vi "KalmanFilterLatencyComp_FindClosestMeasurement.vi"(9 "TimeStamp_Sec":dbl, 11 "in KalmanFilterLatencyCompensator":T1) -> (0 "NotFound":bool, 3 "Index":i32)   [LabVIEW 2019, in "Trajectory_Library.lvlib"]
doc: "An internal function that finds the item in the Past Observer Snapshot list with the timestamp closest to the one passed as an input.\n\nInputs:\n - inKalmanFilterLatencyCompensator -- Data cluster\n - TimeStamp_Sec -- Relative robot timestamp of the item to find (Seconds)\n\nOutputs:\n - Index -- Integer index to the closest entry\n - NotFound -- Boolean, whose value is TRUE if the closest entry was not found."
uses:
  Trajectory_Library.lvlib
  <vilib>/Analysis/Matrix/Datatypes/RealMatrix.ctl
  <vilib>/Analysis/Matrix/NI_Matrix.lvlib
  TypeDef/OBSERVER_SNAPSHOT.ctl
  TypeDef/OBSERVER_SNAP_LIST_ITEM.ctl
  TypeDef/KALMAN_FILTER_LATENCY_COMP.ctl
panel:
  # "<Statess,1>"
  # "<States, States>"
  # "<Inputs, 1>"
  # "<Outputs,  1>"
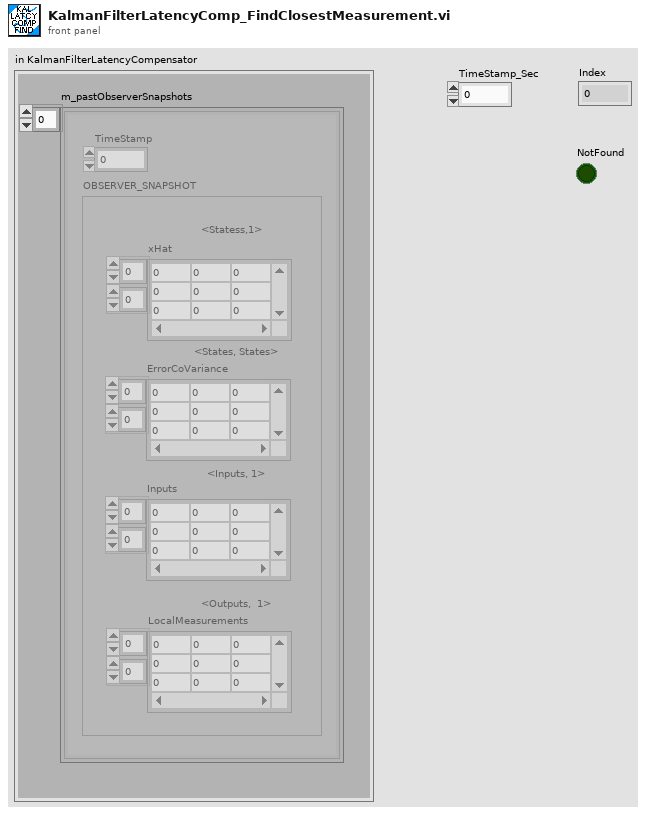
[diagram p1: front panel]
types:
  T1 = typedef "Trajectory_Library.lvlib/KALMAN_FILTER_LATENCY_COMP.ctl" = cluster{"m_pastObserverSnapshots ":T2[]}
  T2 = typedef "Trajectory_Library.lvlib/OBSERVER_SNAP_LIST_ITEM.ctl" = cluster{"TimeStamp":dbl, "OBSERVER_SNAPSHOT":T3}
  T3 = typedef "Trajectory_Library.lvlib/OBSERVER_SNAPSHOT.ctl" = cluster{"ErrorCoVariance":T4, "xHat":T4, "LocalMeasurements":T4, "Inputs":T4}
  T4 = typedef "NI_Matrix.lvlib/RealMatrix.ctl" = dbl[][]
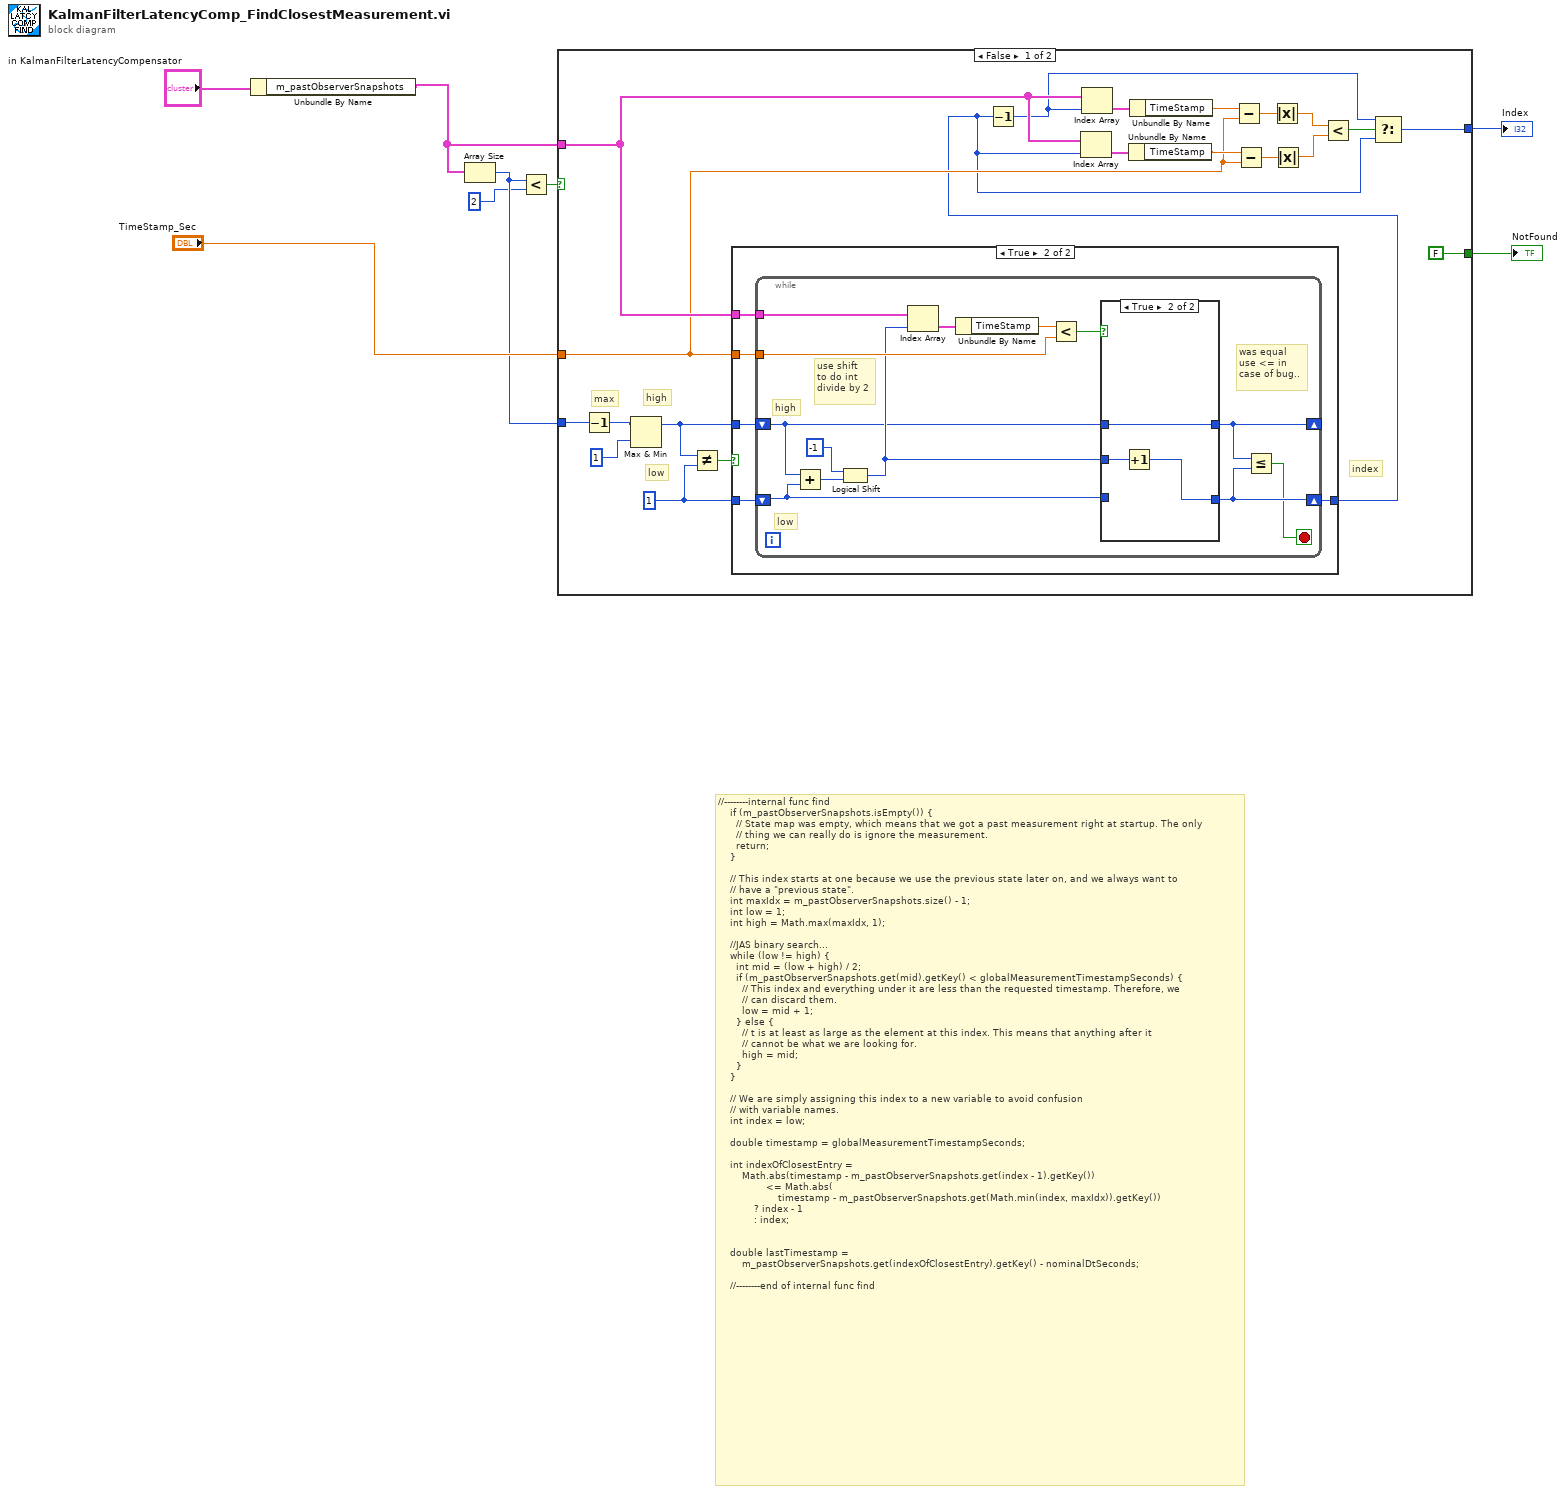
[diagram p0: block diagram]
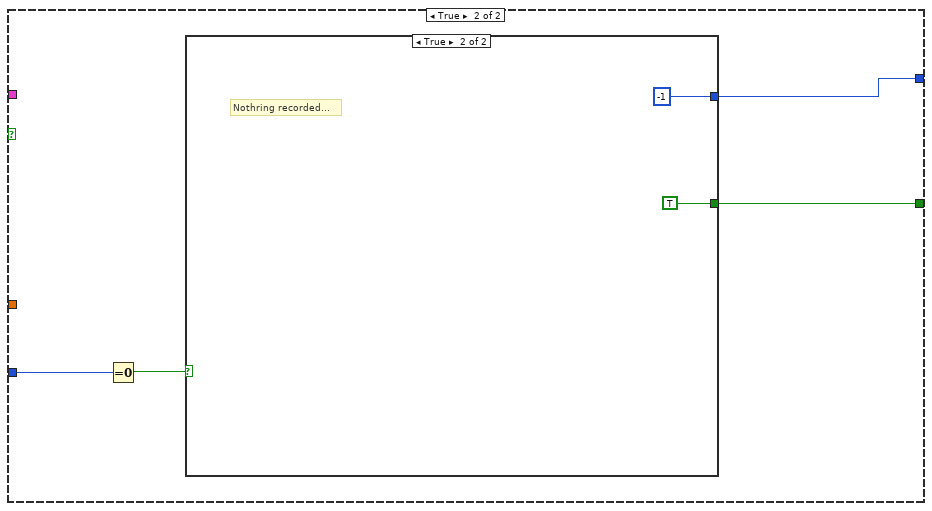
[diagram p4: hidden frame]
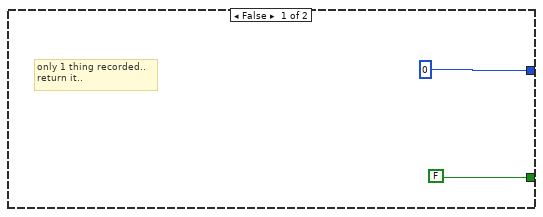
[diagram p5: hidden frame]
diagram:
  # "//--------internal func find\n    if (m_pastObserverSnapshots.isEmpty()) {\n      // State map was empty, which means that we got a past measurement right at startup. The only\n      // thing we can really do is ignore the measurement.\n      return;\n    }\n\n    // This index starts at one because we use the previous state later on, and we always want to\n    // have a \"previous state\".\n    int maxIdx = m_pastObserverSnapshots.size() - 1;\n    int low = 1;\n    int high = Math.max(maxIdx, 1);\n\n    //JAS binary search...\n    while (low != high) {\n      int mid = (low + high) / 2;\n      if (m_pastObserverSnapshots.get(mid).getKey() < globalMeasurementTimestampSeconds) {\n        // This index and everything under it are less than the requested timestamp. Therefore, we\n        // can discard them.\n        low = mid + 1;\n      } else {\n        // t is at least as large as the element at this index. This means that anything after it\n        // cannot be what we are looking for.\n        high = mid;\n      }\n    }\n\n    // We are simply assigning this index to a new variable to avoid confusion\n    // with variable names.\n    int index = low;\n\n    double timestamp = globalMeasurementTimestampSeconds;\n\n    int indexOfClosestEntry =\n        Math.abs(timestamp - m_pastObserverSnapshots.get(index - 1).getKey())\n                <= Math.abs(\n                    timestamp - m_pastObserverSnapshots.get(Math.min(index, maxIdx)).getKey())\n            ? index - 1\n            : index;\n\n\n    double lastTimestamp =\n        m_pastObserverSnapshots.get(indexOfClosestEntry).getKey() - nominalDtSeconds;\n\n    //--------end of internal func find"
  n1 = Unbundle By Name("in KalmanFilterLatencyCompensator") -> ("m_pastObserverSnapshots"=w4:T2[])
  n2 = Array Size(array=w4) -> (size(s)=w2:i32)
  n3 = Less?(x=w2, y=2) -> (x < y?=w3:bool)
  n4 = case shown="False" w3 {
    tunnel: "TimeStamp_Sec" -> [w17 _]
    tunnel: [w9 w54] -> w6
    tunnel: [FALSE w55] -> w5
    tunnel: w2 -> [w27 w57]
    tunnel: w4 -> [w20 _]
    frame False {
      w25 = 1
      # "index"
      # "high"
      # "low"
      # "max"
      n5 = Decrement(x=w27) -> (x-1=w29:i32)
      n6 = Max & Min(x=w29, y=1) -> (max(x,y)=w24:i32)  [unwired: 1 out]
      n7 = Not Equal?(x=w24, y=w25) -> (x != y?=w26:bool)
      n8 = case shown="True" w26 {
        tunnel: w24 -> [_ w35]
        tunnel: w25 -> [w30 w34]
        tunnel: [w30 w31] -> w10
        tunnel: w20 -> [_ w33]
        tunnel: w17 -> [_ w32]
        frame False {
        }
        frame True {
          n9 = while {
            shift-right: [w39] -> w31
            shift-left: w34 -> [w42]
            tunnel: w33 -> [w48]
            tunnel: w32 -> [w45]
            shift-right: [w40] -> _
            shift-left: w35 -> [w41]
            stop <- w38 stop-if-true
            # "was equal\nuse <= in\ncase of bug.."
            # "low"
            # "high"
            # "use shift\nto do int\ndivide by 2"
            n10 = Add(x=w41, y=w42) -> (x+y=w37:i32)
            n11 = Logical Shift(y=-1 ("x"), x=w37) -> (x << y=w43:i32)
            n12 = Index Array(array=w48, index=w43) -> (element=w47:T2)
            n13 = Unbundle By Name(w47) -> ("TimeStamp"=w46:dbl)
            n14 = Less?(x=w46, y=w45) -> (x < y?=w44:bool)
            n15 = case shown="True" w44 {
              tunnel: w43 -> [w49 w53]
              tunnel: [w50 w52] -> w39
              tunnel: w42 -> [w50 _]
              tunnel: [w49 w51] -> w40
              tunnel: w41 -> [_ w51]
              frame False {
              }
              frame True {
                n16 = Increment(x=w53) -> (x+1=w52:i32)
              }
            }
            n17 = Less Or Equal?(x=w40, y=w39) -> (x <= y?=w38:bool)
          }
        }
      }
      n18 = Decrement(x=w10) -> (x-1=w11:i32)
      n19 = Index Array(array=w20, index=w10) -> (element=w21:T2)
      n20 = Index Array(array=w20, index=w11) -> (element=w22:T2)
      n21 = Unbundle By Name(w21) -> ("TimeStamp"=w18:dbl)
      n22 = Unbundle By Name(w22) -> ("TimeStamp"=w19:dbl)
      n23 = Subtract(x=w19, y=w17) -> (x-y=w16:dbl)
      n24 = Subtract(x=w18, y=w17) -> (x-y=w15:dbl)
      n25 = Absolute Value(x=w16) -> (abs(x)=w14:dbl)
      n26 = Absolute Value(x=w15) -> (abs(x)=w13:dbl)
      n27 = Less?(x=w14, y=w13) -> (x < y?=w12:bool)
      n28 = Select(t=w11, s=w12, f=w10) -> (s? t:f=w9:i32)
    }
    frame True {
      n29 = Equal To 0?(x=w57) -> (x = 0?=w56:bool)
      n30 = case shown="True" w56 {
        tunnel: [FALSE TRUE] -> w55
        tunnel: [0 -1] -> w54
        frame False {
          # "only 1 thing recorded..\nreturn it.."
        }
        frame True {
          # "Nothring recorded..."
        }
      }
    }
  }
  "NotFound" <- w5
  "Index" <- w6
